vi "HAL camera initialize.vi"() -> (0 "error out":errorcluster)   [LabVIEW 2011]
uses:
  ixon1024/HAL Camera specifications globals.vi
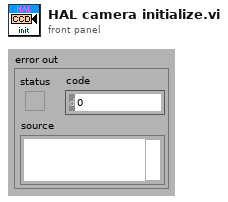
[diagram p1: front panel]
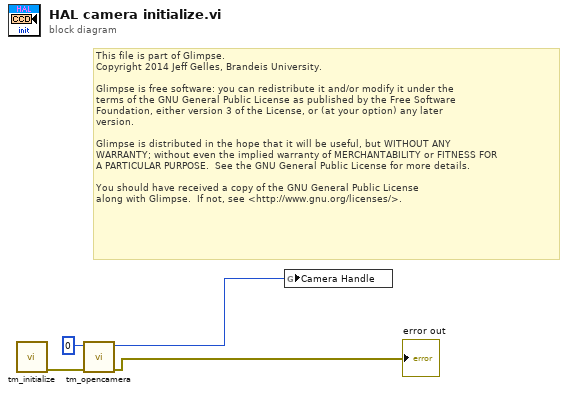
[diagram p0: block diagram]
diagram:
  # "This file is part of Glimpse. \nCopyright 2014 Jeff Gelles, Brandeis University.    \n\nGlimpse is free software: you can redistribute it and/or modify it under the \nterms of the GNU General Public License as published by the Free Software \nFoundation, either version 3 of the License, or (at your option) any later \nversion.\n\nGlimpse is distributed in the hope that it will be useful, but WITHOUT ANY \nWARRANTY; without even the implied warranty of MERCHANTABILITY or FITNESS FOR \nA PARTICULAR PURPOSE.  See the GNU General Public License for more details.\n\nYou should have received a copy of the GNU General Public License\nalong with Glimpse.  If not, see <http://www.gnu.org/licenses/>."
  n1 = call <userlib>:"tm_initialize.vi"() -> ("error out"=w3:errorcluster)  [unwired: 10 in, 1 out]
  n2 = call <userlib>:"tm_opencamera.vi"("error in (no error)"=w3, "Camera Index"=u32 0) -> ("error out"=→"error out":errorcluster, "Handle out"=w2:u32)  [unwired: 8 in]
  n3 = global write "HAL Camera specifications globals.vi" "Camera Handle"(w2) -> ()
